vi "upload_from_file.vi"(1 "Spreadsheet path":path) -> (0 "Cell Settings Array 4":T1=[{"Measure?"=TRUE, "Area (cm^2)"=0.0, "Cell Label"="", "Cell Description"="", "Time between scans (s)"=0.0, "Cell Position"=1, "Scan settings in queue"=0, "Sample holder"=4.0, "User name"=""}, {"Measure?"=TRUE, "Area (cm^2)"=0.0, "Cell Label"="", "Cell Description"="", "Time between scans (s)"=0.0, "Cell Position"=2, "Scan settings in queue"=0, "Sample holder"=4.0, "User name"=""}, {"Measure?"=TRUE, "Area (cm^2)"=0.0, "Cell Label"="", "Cell Description"="", "Time between scans (s)"=0.0, "Cell Position"=3, "Scan settings in queue"=0, "Sample holder"=4.0, "User name"=""}, {"Measure?"=TRUE, "Area (cm^2)"=0.0, "Cell Label"="", "Cell Description"="", "Time between scans (s)"=0.0, "Cell Position"=4, "Scan settings in queue"=0, "Sample holder"=4.0, "User name"=""}, {"Measure?"=TRUE, "Area (cm^2)"=0.0, "Cell Label"="", "Cell Description"="", "Time between scans (s)"=0.0, "Cell Position"=5, "Scan settings in queue"=0, "Sample holder"=4.0, "User name"=""}, {"Measure?"=TRUE, "Area (cm^2)"=0.0, "Cell Label"="", "Cell Description"="", "Time between scans (s)"=0.0, "Cell Position"=6, "Scan settings in queue"=0, "Sample holder"=4.0, "User name"=""}, {"Measure?"=TRUE, "Area (cm^2)"=0.0, "Cell Label"="", "Cell Description"="", "Time between scans (s)"=0.0, "Cell Position"=7, "Scan settings in queue"=0, "Sample holder"=4.0, "User name"=""}, {"Measure?"=TRUE, "Area (cm^2)"=0.0, "Cell Label"="", "Cell Description"="", "Time between scans (s)"=0.0, "Cell Position"=8, "Scan settings in queue"=0, "Sample holder"=4.0, "User name"=""}, {"Measure?"=TRUE, "Area (cm^2)"=0.0, "Cell Label"="", "Cell Description"="", "Time between scans (s)"=0.0, "Cell Position"=9, "Scan settings in queue"=0, "Sample holder"=4.0, "User name"=""}, {"Measure?"=TRUE, "Area (cm^2)"=0.0, "Cell Label"="", "Cell Description"="", "Time between scans (s)"=0.0, "Cell Position"=10, "Scan settings in queue"=0, "Sample holder"=4.0, "User name"=""}, {"Measure?"=TRUE, "Area (cm^2)"=0.0, "Cell Label"="", "Cell Description"="", "Time between scans (s)"=0.0, "Cell Position"=11, "Scan settings in queue"=0, "Sample holder"=4.0, "User name"=""}, {"Measure?"=TRUE, "Area (cm^2)"=0.0, "Cell Label"="", "Cell Description"="", "Time between scans (s)"=0.0, "Cell Position"=12, "Scan settings in queue"=0, "Sample holder"=4.0, "User name"=""}, {"Measure?"=TRUE, "Area (cm^2)"=0.0, "Cell Label"="", "Cell Description"="", "Time between scans (s)"=0.0, "Cell Position"=13, "Scan settings in queue"=0, "Sample holder"=4.0, "User name"=""}, {"Measure?"=TRUE, "Area (cm^2)"=0.0, "Cell Label"="", "Cell Description"="", "Time between scans (s)"=0.0, "Cell Position"=14, "Scan settings in queue"=0, "Sample holder"=4.0, "User name"=""}, {"Measure?"=TRUE, "Area (cm^2)"=0.0, "Cell Label"="", "Cell Description"="", "Time between scans (s)"=0.0, "Cell Position"=15, "Scan settings in queue"=0, "Sample holder"=4.0, "User name"=""}, {"Measure?"=TRUE, "Area (cm^2)"=0.0, "Cell Label"="", "Cell Description"="", "Time between scans (s)"=0.0, "Cell Position"=16, "Scan settings in queue"=0, "Sample holder"=4.0, "User name"=""}] {"Scan settings in queue" items=["Standard"]})   [LabVIEW 2011]
uses:
  Typedefs/Cell details array.ctl
  Typedefs/Cell details cluster.ctl
  <vilib>/Utility/file.llb/Read From Spreadsheet File (string).vi
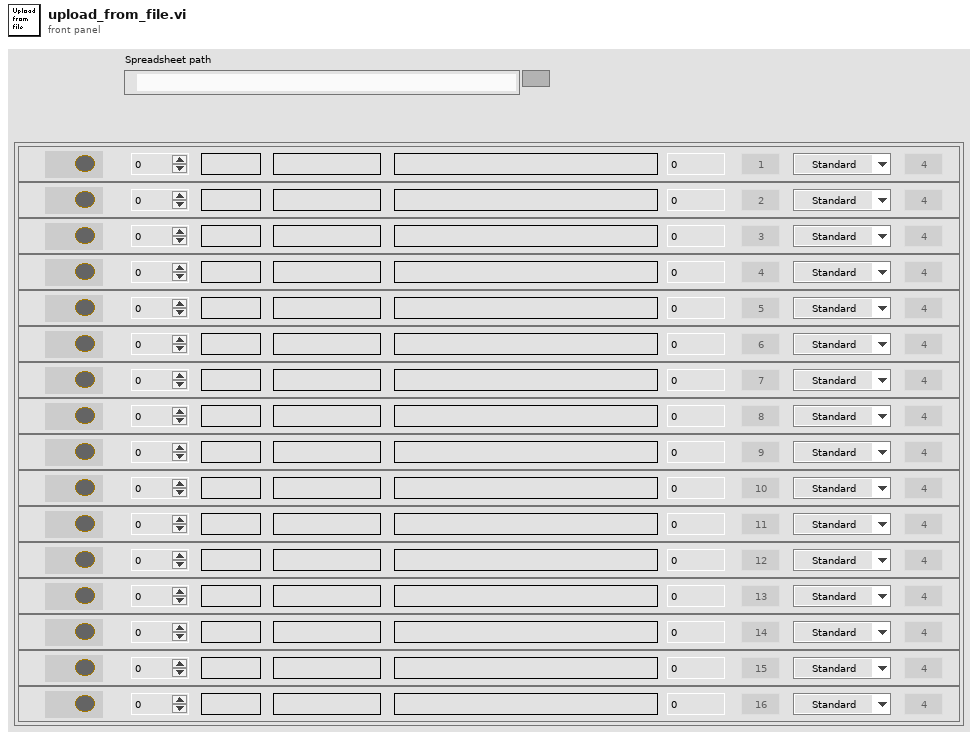
[diagram p1: front panel]
types:
  T1 = typedef "Cell details array.ctl" = T2[]
  T2 = typedef "Cell details cluster.ctl" = cluster{"Measure?":bool, "Area (cm^2)":dbl, "Cell Label":string, "Cell Description":string, "Time between scans (s)":dbl, "Cell Position":i32, "Scan settings in queue":u16, "Sample holder":dbl, "User name":string}
  T3 = cluster{"Measure?":bool, "Area (cm^2)":dbl, "Cell Label":string, "Cell Description":string, "Time between scans (min)":dbl, "Cell Position":i32, "Scan settings in queue":u16, "Sample Holder":dbl, "User Name":string}
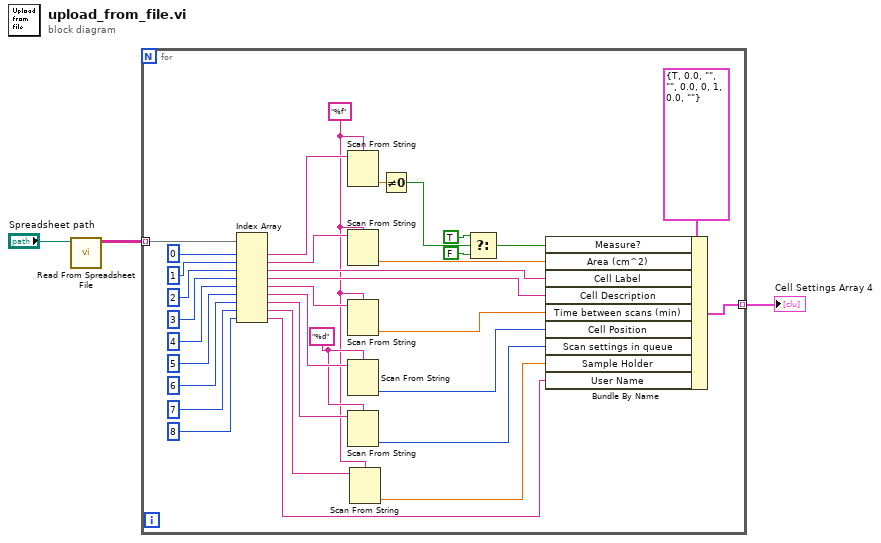
[diagram p0: block diagram]
diagram:
  n1 = call-poly <vilib>:"Read From Spreadsheet File.vi"("file path (dialog if empty)"="Spreadsheet path") -> ("all rows"=w2:string[][])  [unwired: 6 in, 4 out]
  n2 = for {
    tunnel: w2 -> [w36] mode=indexing
    tunnel: [w35] -> w1 mode=indexing
    w9 = "%d" ("format string")
    w8 = "%f" ("format string")
    n3 = Index Array(array=w36, index #1=0 ("index"), index #2=1 ("index"), index #3=2 ("index"), index #4=3 ("index"), index #5=4 ("index"), index #6=5 ("index"), index #7=6 ("index"), index #8=7 ("index"), index #9=8 ("index")) -> (element #1=w29:string, element #2=w23:string, element #3=w21:string, element #4=w20:string, element #5=w19:string, element #6=w16:string, element #7=w13:string, element #8=w7:string, element #9=w4:string)
    n4 = Scan From String(format string=w8, input string=w29) -> (output 1=w28:dbl)  [unwired: 3 in, 3 out]
    n5 = Scan From String(format string=w8, input string=w23) -> (output 1=w22:dbl)  [unwired: 3 in, 3 out]
    n6 = Scan From String(format string=w8, input string=w19) -> (output 1=w18:dbl)  [unwired: 3 in, 3 out]
    n7 = Scan From String(format string=w9, input string=w16) -> (output 1=w15:i32)  [unwired: 3 in, 3 out]
    n8 = Scan From String(format string=w9, input string=w13) -> (output 1=w11:i32)  [unwired: 3 in, 3 out]
    n9 = Scan From String(format string=w8, input string=w7) -> (output 1=w6:dbl)  [unwired: 3 in, 3 out]
    n10 = Not Equal To 0?(x=w28) -> (x != 0?=w27:bool)
    n11 = Select(t=TRUE, s=w27, f=FALSE) -> (s? t:f=w24:bool)
    n12 = Bundle By Name(cluster=T3 {"Measure?"=TRUE, "Area (cm^2)"=0.0, "Cell Label"="", "Cell Description"="", "Time between scans (min)"=0.0, "Cell Position"=0, "Scan settings in queue"=1, "Sample Holder"=0.0, "User Name"=""} ("Cluster"), "Measure?"=w24, "Area (cm^2)"=w22, "Cell Label"=w21, "Cell Description"=w20, "Time between scans (min)"=w18, "Cell Position"=w15, "Scan settings in queue"=w11, "Sample Holder"=w6, "User Name"=w4) -> (w35:T3)
  }
  "Cell Settings Array 4" <- w1
